vi "Read CSV File and Select Clock.vi"() -> ()   [LabVIEW 2020]
uses:
  <vilib>/Utility/sysdir.llb/System Directory Type.ctl
  <vilib>/Utility/file.llb/Read Delimited Spreadsheet (string).vi
  Selected Clock(Global Variable).vi
panel:
  out "Selected Clock":timestamp format="%<%X\n%x>T"
  in  "stop":bool
  in  "Select Clock":i32=1 min=1
  out "Table Control":string[][](table)=[["# of Clocks", "Day", "Alarm time"], ["1", "5.05.2020", "07:30:00"], ["2", "5.05.2020", "08:00:00"], ["3", "5.05.2020", "08:30:00"], ["4", "5.05.2020", "09:00:00"], ["5", "5.05.2020", "09:30:00"], ["6", "5.05.2020", "10:00:00"], ["7", "5.05.2020", "10:30:00"], ["8", "5.05.2020", "11:00:00"], ["9", "5.05.2020", "11:30:00"], ["10", "5.05.2020", "12:00:00"], ["11", "5.05.2020", "12:30:00"], ["12", "5.05.2020", "13:00:00"], ["13", "5.05.2020", "13:30:00"], ["14", "5.05.2020", "14:00:00"], ["15", "5.05.2020", "14:30:00"], ["16", "5.05.2020", "15:00:00"], ["17", "5.05.2020", "15:30:00"], ["18", "5.05.2020", "16:00:00"], ["19", "5.05.2020", "16:30:00"], ["20", "5.05.2020", "17:00:00"]]
  # "Please select the number of the that clock you want to work with in the next step then you can stop the program and run  Alarm Clock.VI"
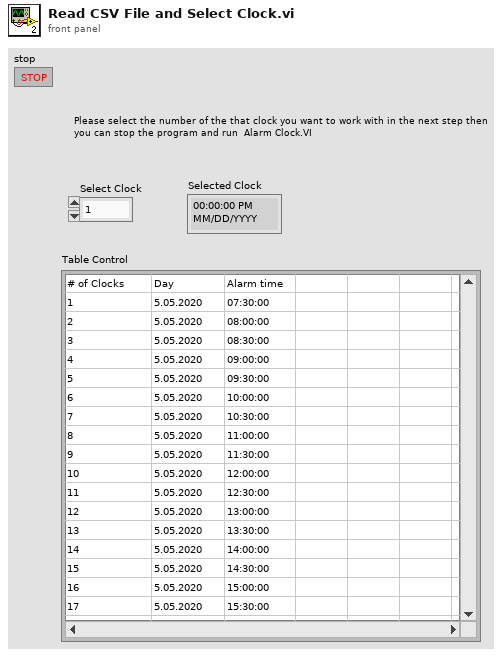
[diagram p1: front panel]
types:
  T1 = typedef "System Directory Type.ctl" = i32
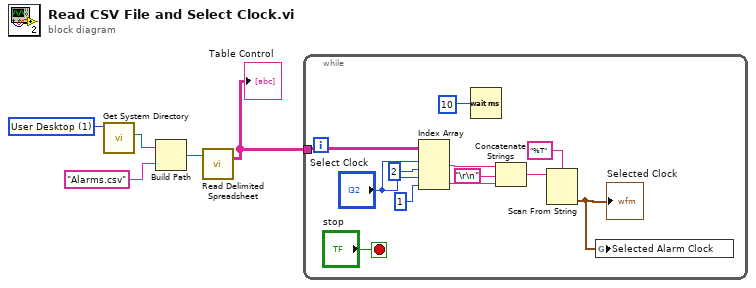
[diagram p0: block diagram]
diagram:
  w5 = T1 1 items=["User Home"=0, "User Desktop"=1, "User Documents"=2, "User Application Data"=3, "User Preferences"=4, "User Temporary"=5, "Public Documents"=6, "Public Application Data"=7, "Public Preferences"=8, "Public Cache"=13, "System Core Libraries"=9, "System Installed Libraries"=10, "Application Files"=11, "Boot Volume Root"=12] ("system directory type")
  n1 = call <vilib>:"Get System Directory.vi"("system directory type"=w5) -> ("system directory"=w4:path)  [unwired: 10 in]
  n2 = Build Path(base path=w4, name or relative path="Alarms.csv") -> (appended path=w3:path)
  n3 = call-poly <vilib>:"Read Delimited Spreadsheet.vi"("file path (dialog if empty)"=w3) -> ("all rows"=w1:string[][])  [unwired: 9 in, 5 out]
  "Table Control" <- w1
  n4 = while {
    tunnel: w1 -> [w16]
    stop <- "stop" stop-if-true
    n5 = Index Array(array=w16, index (row) #1="Select Clock", index (col) #1=2 ("disabled index (col)"), index (row) #2="Select Clock", index (col) #2=1 ("disabled index (col)")) -> (element #1=w11:string, element #2=w9:string)
    n6 = Wait (ms)(milliseconds to wait=u32 10) -> ()  [unwired: 1 out]
    n7 = Concatenate Strings(w11, "\r\n", w9) -> (w7:string)
    n8 = Scan From String(format string="%T", input string=w7) -> (output 1=w6:timestamp)  [unwired: 3 in, 3 out]
    "Selected Clock" <- w6
    n9 = global write "Selected Clock(Global Variable).vi" "Selected Alarm Clock"(w6) -> ()
  }
